vi "ComboBoxDisptxt.vi"() -> (2 "cadena":string[](array[string]))   [LabVIEW 2016]
uses:
  <vilib>/Utility/file.llb/Read Delimited Spreadsheet (string).vi
panel:
  out "all rows":string[][](array[string])
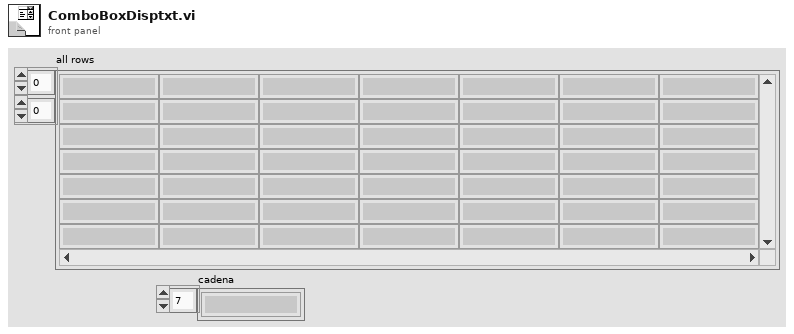
[diagram p1: front panel]
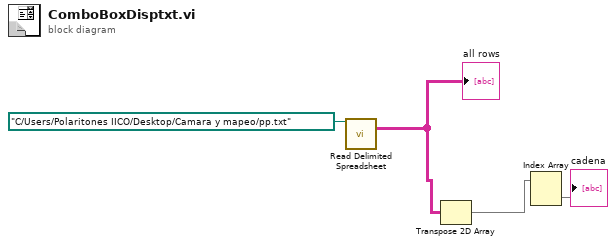
[diagram p0: block diagram]
diagram:
  n1 = call-poly <vilib>:"Read Delimited Spreadsheet.vi"("file path (dialog if empty)"=path "C:/Users/Polaritones IICO/Desktop/Camara y mapeo/pp.txt") -> ("all rows"=w2:string[][])  [unwired: 9 in, 5 out]
  "all rows" <- w2
  n2 = Transpose 2D Array(2D array=w2) -> (transposed array=w1:string[][])
  n3 = Index Array(array=w1) -> (element=→"cadena":string[])  [unwired: 2 in]
